vi "GetFSSOuterTunnelReference.vi"(8 "error in":errorcluster, 11 "Tunnel in":refnum<class "FlatSequenceOuterTunnel.lvclass">) -> (0 "error out":errorcluster, 1 "reference out":refnum<vi>, 3 "Tunnel out":refnum<class "FlatSequenceOuterTunnel.lvclass">)   [LabVIEW 2014, in "Raspberry Pi Compatible Compiler for LabVIEW.lvlib" / "FlatSequenceOuterTunnel.lvclass"]
uses:
  FlatSequenceOuterTunnel.lvclass
  Generic/Generic.lvclass
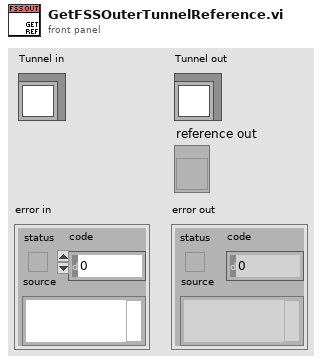
[diagram p1: front panel]
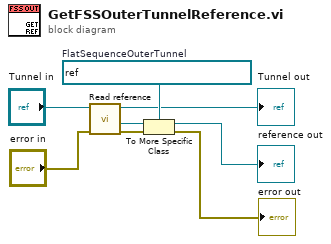
[diagram p0: block diagram]
diagram:
  w8 = refnum<vi> refnum  # FlatSequenceOuterTunnel
  n1 = call "Read reference.vi"("error in"="error in", "GObject in"="Tunnel in") -> ("error out"=w7:errorcluster, "reference"=w6:refnum<vi>, "GObject out"=→"Tunnel out":refnum<class "FlatSequenceOuterTunnel.lvclass">)  [unwired: 5 in]
  n2 = To More Specific Class(target class=w8, reference=w6, error in=w7) -> (specific class reference=→"reference out":refnum<vi>, error out=→"error out":errorcluster)
